vi "Global_Application Path.vi"(1 "Use ExeFilePath":bool) -> (0 "程序路径":path)   [LabVIEW 2011]
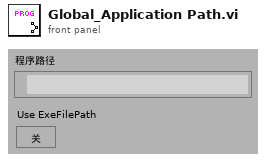
[diagram p1: front panel]
types:
  T1 = enum32{"invalid app kind", "Development System", "Run Time System", "Student Edition", "Embedded LabVIEW", "Evaluation", "Custom"}
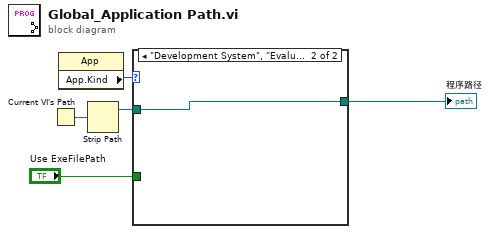
[diagram p0: block diagram]
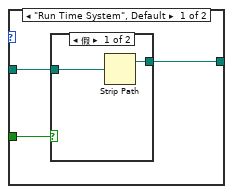
[diagram p2: hidden frame]
diagram:
  n1 = Current VI's Path() -> (path=w1:path)
  n2 = property class="App"() -> ("App.Kind"=w5:T1)  [unwired: 2 in, 2 out]
  n3 = Strip Path(path=w1) -> (stripped path=w3:path)  [unwired: 1 out]
  n4 = case shown="\"Development System\", \"Evaluation\"" w5 {
    tunnel: w3 -> [w8 w12]
    tunnel: [w6 w12] -> w4
    tunnel: "Use ExeFilePath" -> [w7 _]
    frame "Run Time System", Default {
      n5 = case shown="假" w7 {
        tunnel: w8 -> [w10 w11]
        tunnel: [w9 w11] -> w6
        frame False {
          n6 = Strip Path(path=w10) -> (stripped path=w9:path)  [unwired: 1 out]
        }
        frame True {
        }
      }
    }
    frame "Development System", "Evaluation" {
    }
  }
  "程序路径" <- w4
